vi "Write PLC Settings.vi"(8 "error in (no error)":errorcluster, 10 "PLC Settings":T1={"Port"="", "BaudRate"=9600, "Wakeup Signal Address "=0.0, "Acquisiton Address"=0.0, "Acknowledgement Address"=0.0, "Sleep Address"=0.0}, 11 "Controller in":refnum<class "Controller.lvclass">) -> (0 "error out":errorcluster, 3 "Controller out":refnum<class "Controller.lvclass">)   [LabVIEW 2022 SP3, in "Controller.lvlib" / "Controller.lvclass"]
uses:
  Controller.lvclass
  Typedefs/PLC Settings.ctl
  Controller.lvclass/Controller.ctl
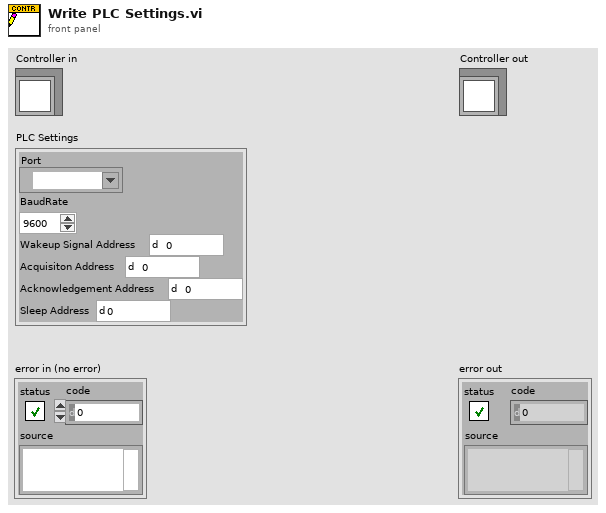
[diagram p1: front panel]
types:
  T1 = typedef "PLC Settings.ctl" = cluster{"Port":refnum<visa-resource-name>, "BaudRate":u32, "Wakeup Signal Address ":dbl, "Acquisiton Address":dbl, "Acknowledgement Address":dbl, "Sleep Address":dbl}
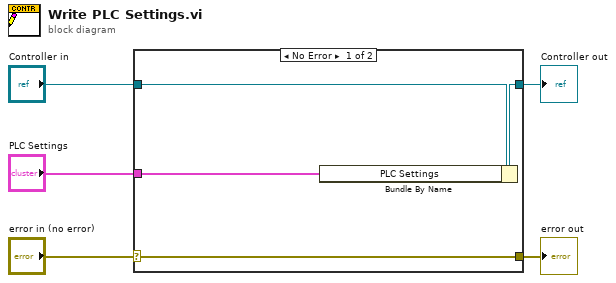
[diagram p0: block diagram]
diagram:
  n1 = case shown="No Error" "error in (no error)" {
    selector: "error in (no error)" -> [w9 w10]
    tunnel: [w9 w10] -> w4
    tunnel: [w7 w11] -> w2
    tunnel: "Controller in" -> [w8 w11]
    tunnel: "PLC Settings" -> [w6 _]
    frame No Error {
      n2 = Bundle By Name(cluster=w8, "PLC Settings"=w6) -> (w7:refnum<class "Controller.lvclass">)
    }
    frame Error {
    }
  }
  "error out" <- w4
  "Controller out" <- w2
